vi "Actor Core.vi"(8 "error in":errorcluster, 11 "Measurement Timer in":refnum<class "Measurement Timer.lvclass">) -> (0 "error out":errorcluster, 3 "Actor out":refnum<class "Actor.lvclass">)   [LabVIEW 2015, in "Measurement Timer.lvclass"]
doc: "(<B>Filename</B>: Actor Framework.lvlib:Actor.lvclass:Actor Core.vi)\n\nReceives messages to the actor, reacts to them, and initiates any error handling that may shut the actor down.\n\nDescendant classes may override this VI to append parallel tasks for the actor to complete while it handles messages. Overrides use the Call Parent Method node."
uses:
  Measurement Timer.lvclass
  <vilib>/ActorFramework/Actor/Actor.lvclass
  Timer Parameters.ctl
  Log time.ctl
  Mag Lab Measurement/Mag Lab Measurement.lvclass
panel:
  in  "Parameters":T1={"millisecond multiple"=1000, "Time reference"=enum."Relative"}
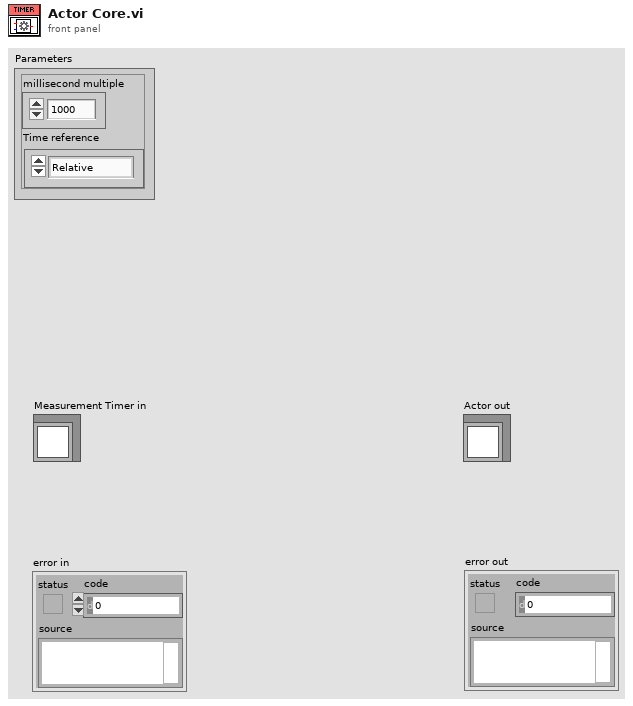
[diagram p1: front panel]
types:
  T1 = typedef "Timer Parameters.ctl" = cluster{"millisecond multiple":u32, "Time reference":T2}
  T2 = typedef "Log time.ctl" = enum16{"Relative", "Absolute", "Do not log"}
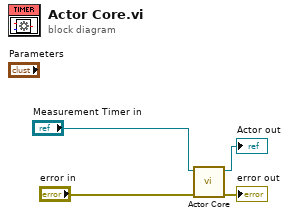
[diagram p0: block diagram]
diagram:
  n1 = call-parent "Actor Core.vi"("error in"="error in", "Mag Lab Measure Base in"="Measurement Timer in") -> ("error out"=→"error out":errorcluster, "Actor out"=→"Actor out":refnum<class "Actor.lvclass">)  [unwired: 8 in]
